vi "dataUnpackString.vi"(8 "errorIn":errorcluster, 11 "data":variant) -> (0 "errorOut":errorcluster, 3 "String":string)   [LabVIEW 2017]
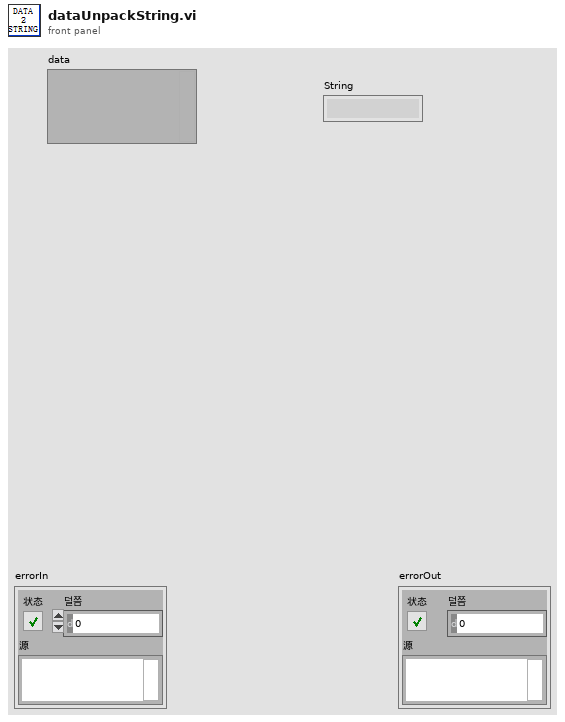
[diagram p1: front panel]
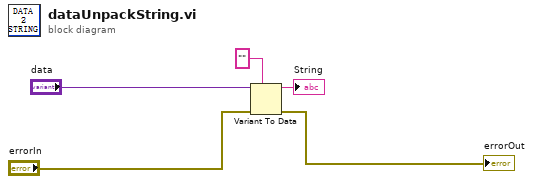
[diagram p0: block diagram]
diagram:
  n1 = Variant To Data(error in="errorIn", type="", Variant="data") -> (data=→"String":string, error out=→"errorOut":errorcluster)
